vi "Car-Wash.vi"() -> ()   [LabVIEW 2017]
panel:
  out "Enum 2":enum16{"ECO", "DEL"}(ring)
  in  "Enum":enum16{"DEL", "ECO"}(ring)
  in  "MWP 2":bool
  in  "?":bool
  out "output cluster":cluster{bool, bool}
  in  "Economy Wash":bool
  in  "Deluxe Wash":bool
  in  "MWP":bool
  out "Vehicle Out of Position":bool=TRUE
  out "Air Dry":bool
  out "Clear Water Rinse":bool
  out "Main High Press. Wash":bool
  out "Soap Application":bool
  out "Under body Wash":bool
  in  "ADP":bool
  in  "UBW":bool
  # "AUTOMATED CAR WASH"
  # "Purchase Selection"
  # "Car Wash Indicators"
  # "Car Wash Simulation Switches"
  # "Underbody wash\nposition \nSwitch"
  # "Main Wash \nPosition \nSwitch"
  # "Air Dry\nPosition\nSwitch"
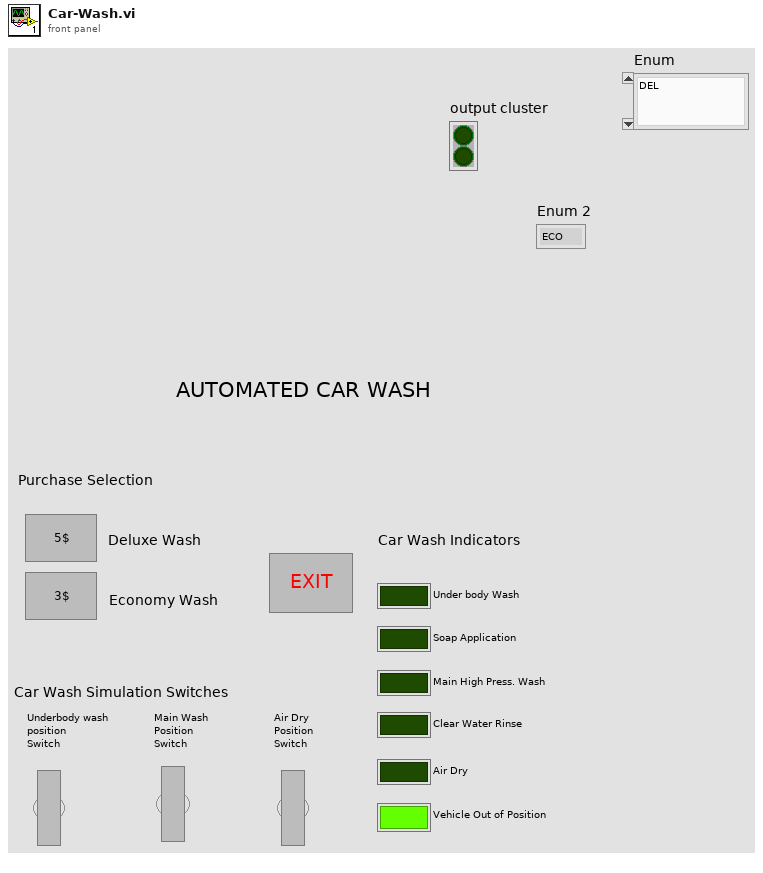
[diagram p1: front panel]
types:
  T1 = enum8{"Enabled", "Disabled", "Disabled and Grayed Out"}
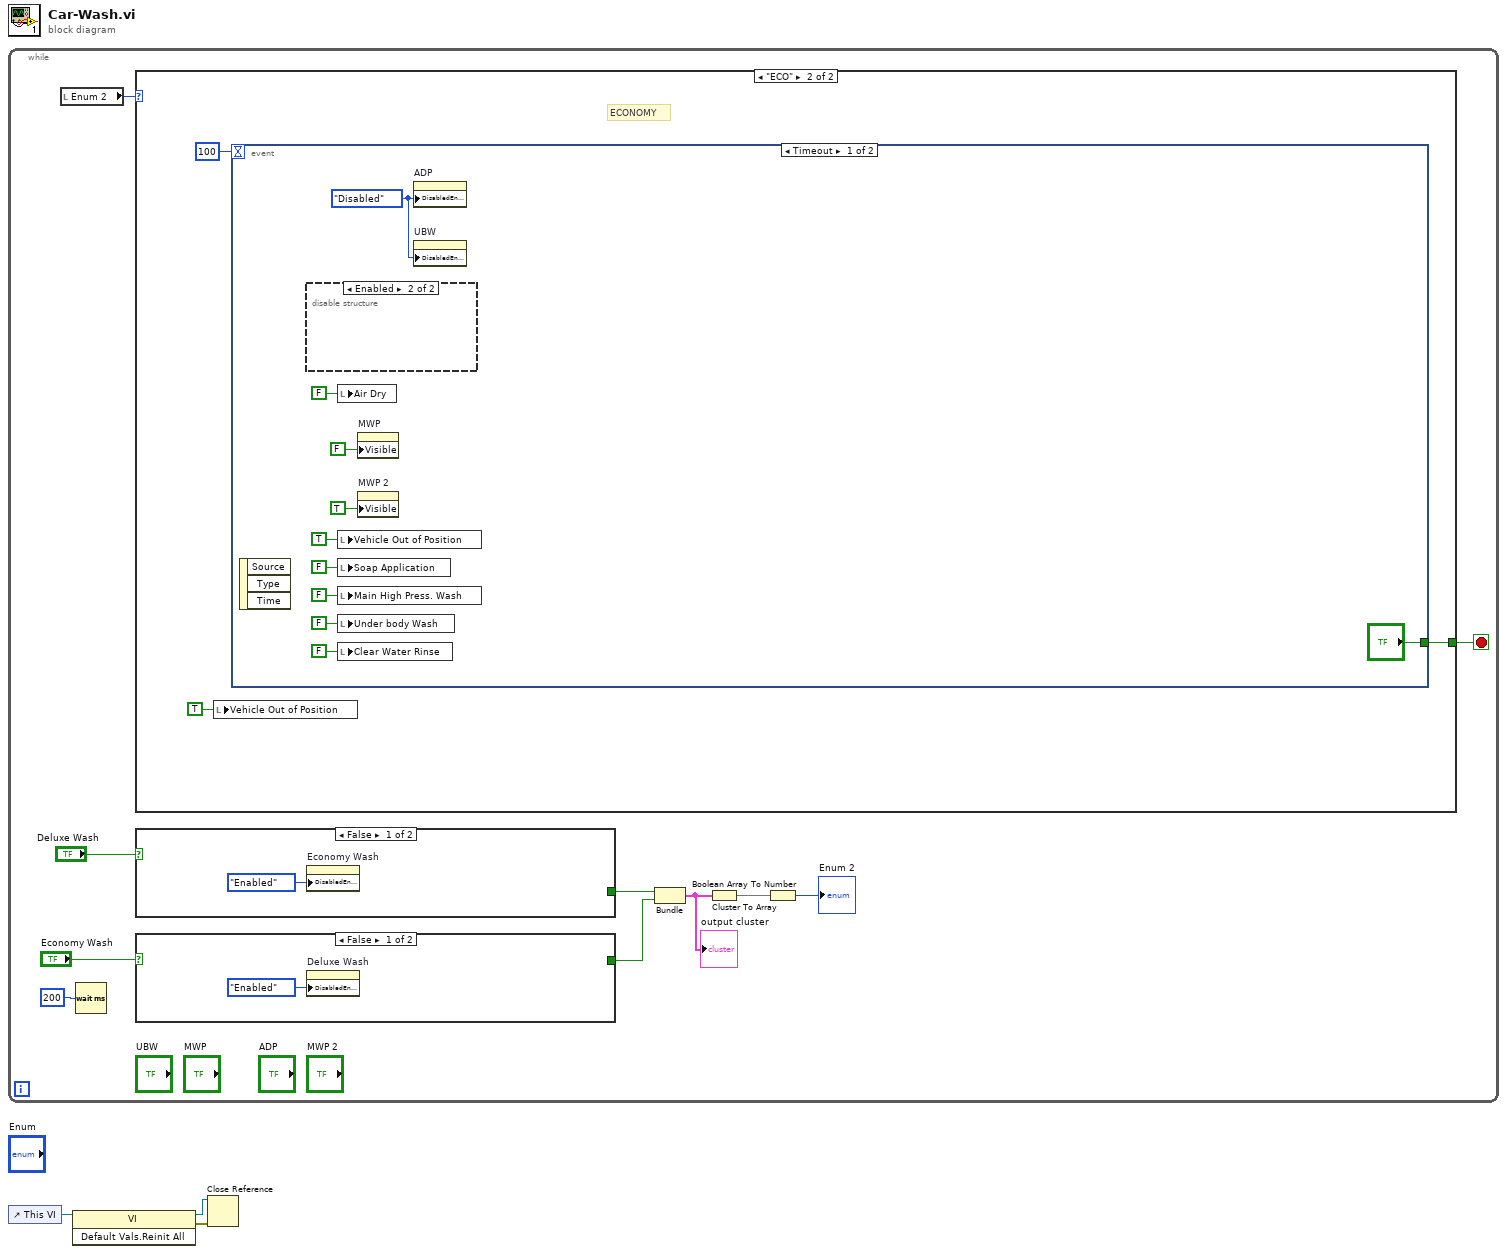
[diagram p0: block diagram]
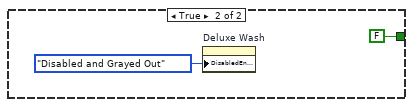
[diagram p2: hidden frame]
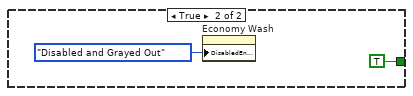
[diagram p3: hidden frame]
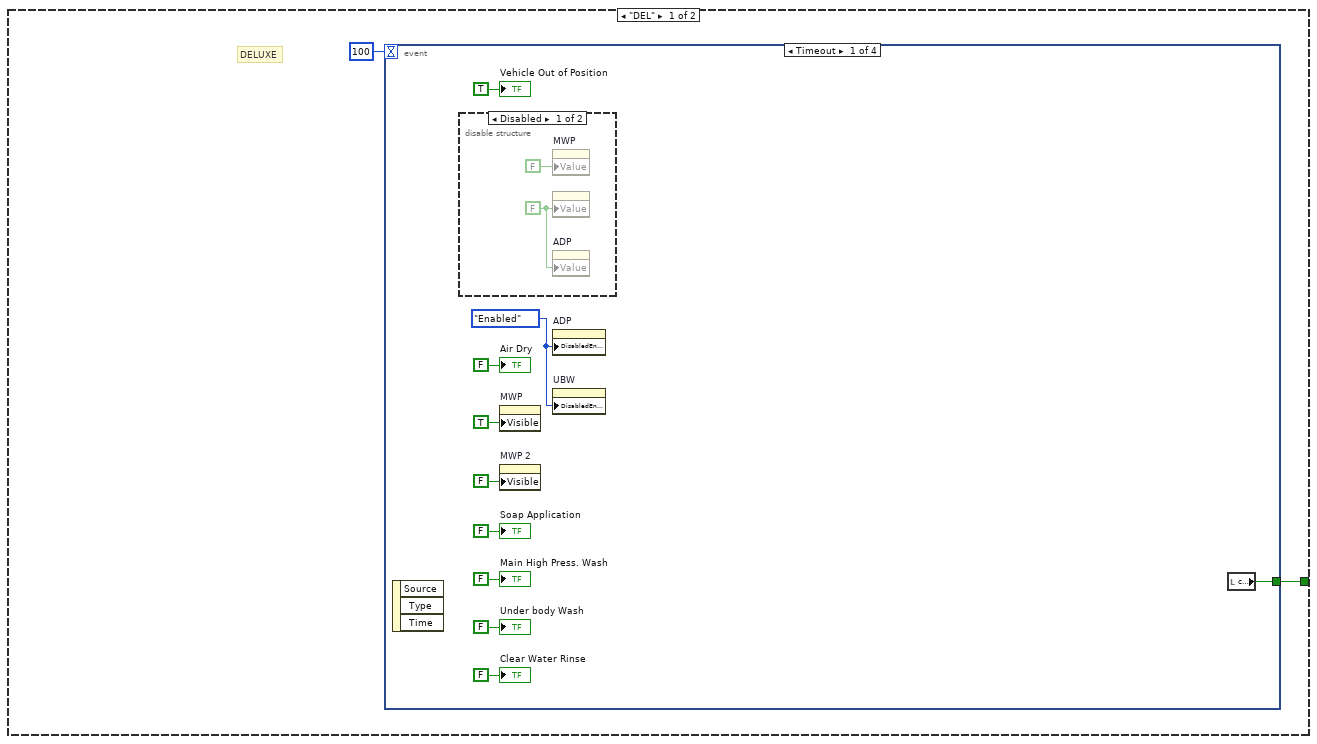
[diagram p4: hidden frame]
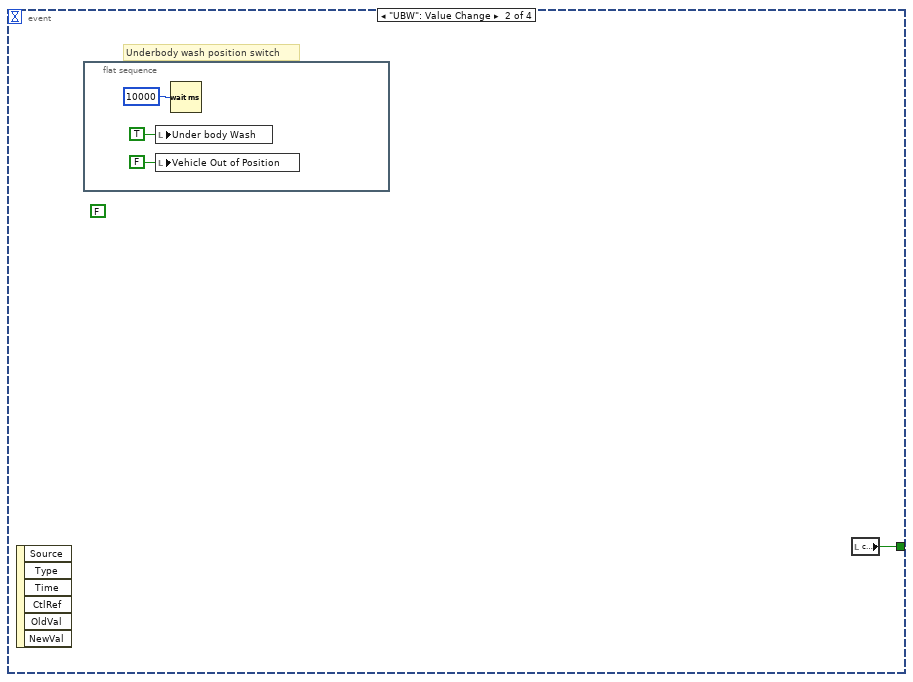
[diagram p6: hidden frame]
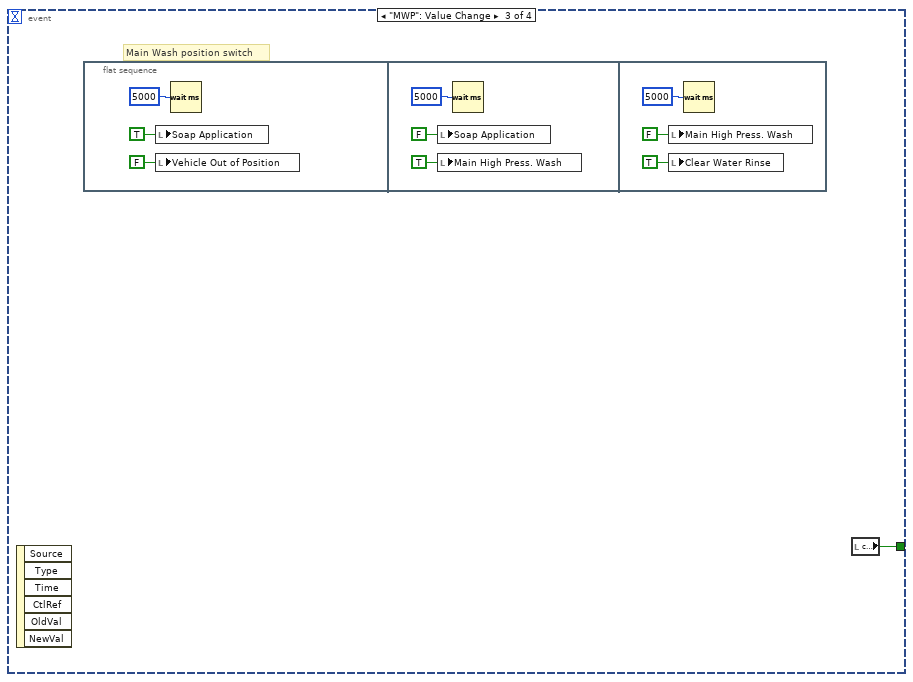
[diagram p7: hidden frame]
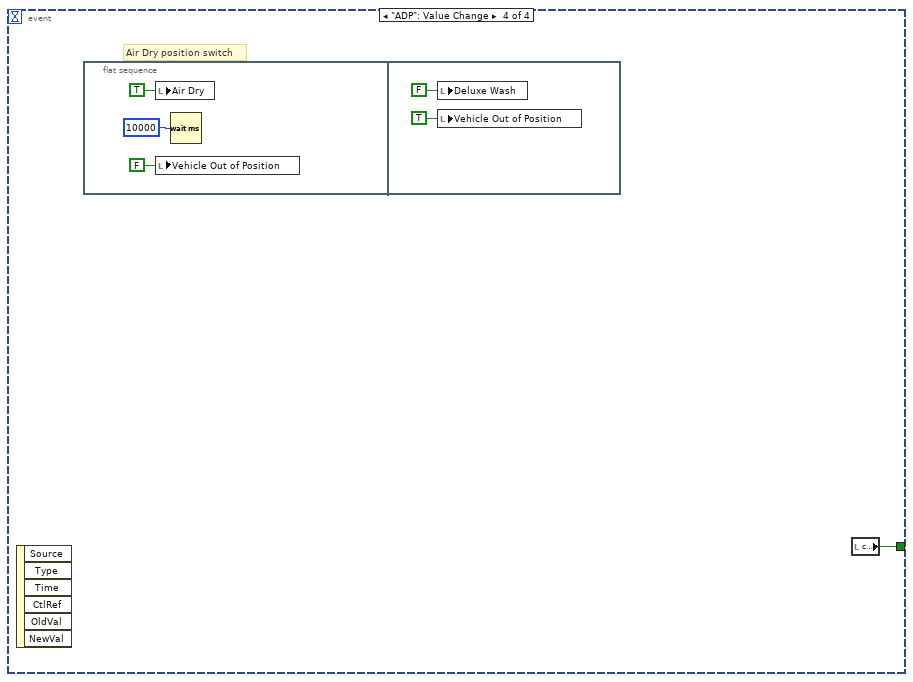
[diagram p8: hidden frame]
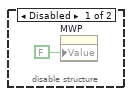
[diagram p9: hidden frame]
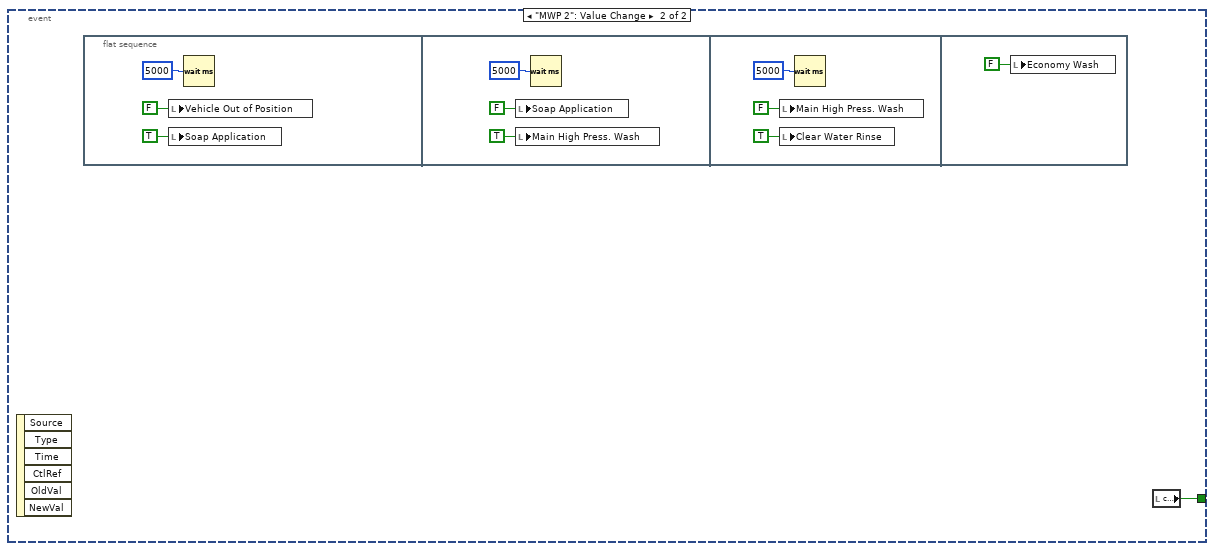
[diagram p10: hidden frame]
diagram:
  n1 = while {
    stop <- w12 stop-if-true
    n2 = local read "Enum 2"() -> (w4:enum16{"ECO", "DEL"})
    n3 = Wait (ms)(milliseconds to wait=u32 200) -> ()  [unwired: 1 out]
    n4 = case shown="\"ECO\"" w4 {
      tunnel: [w20 w54] -> w12
      frame "DEL" {
        # "DELUXE"
        n5 = event shown="[0] Timeout" {
          selector: _ -> [_ _ _ _]
          dyn-events: _ -> [_ _ _ _]
          timeout: 100 -> [_ _ _ _]
          tunnel: [w24 w34 w38 w48] -> w20
          event Timeout {
            w26 = T1."Enabled" ("Disabled")
            n6 = event-data() -> ()  [unwired: 1 in, 3 out]
            n7 = disable-structure shown="Disabled" {
              frame Disabled {
                w33 = FALSE
                n8 = property on="MWP" class="Bool"("Value"=FALSE) -> ()  [unwired: 2 in, 2 out]
                n9 = property on="UBW" class="Bool"("Value"=w33) -> ()  [unwired: 2 in, 2 out]
                n10 = property on="ADP" class="Bool"("Value"=w33) -> ()  [unwired: 2 in, 2 out]
              }
              frame Enabled {
              }
            }
            n11 = property on="MWP" class="Bool"("Visible"=TRUE) -> ()  [unwired: 2 in, 2 out]
            n12 = property on="MWP 2" class="Bool"("Visible"=FALSE) -> ()  [unwired: 2 in, 2 out]
            n13 = property on="ADP" class="Bool"("DisabledEnum"=w26) -> ()  [unwired: 2 in, 2 out]
            n14 = property on="UBW" class="Bool"("DisabledEnum"=w26) -> ()  [unwired: 2 in, 2 out]
            n15 = local read item#12() -> (w24:bool)
            "Air Dry" <- FALSE
            "Vehicle Out of Position" <- TRUE
            "Clear Water Rinse" <- FALSE
            "Under body Wash" <- FALSE
            "Main High Press. Wash" <- FALSE
            "Soap Application" <- FALSE
          }
          event "UBW": Value Change {
            (unwired) FALSE
            # "Underbody wash position switch"
            n16 = event-data() -> ()  [unwired: 1 in, 6 out]
            n17 = flat-sequence {
              frame #0 {
                n18 = local write "Under body Wash"(TRUE ("Under body Wash")) -> ()
                n19 = local write "Vehicle Out of Position"(FALSE ("Vehicle Out of Position")) -> ()
                n20 = Wait (ms)(milliseconds to wait=u32 10000) -> ()  [unwired: 1 out]
              }
            }
            n21 = local read item#12() -> (w34:bool)
          }
          event "MWP": Value Change {
            # "Main Wash position switch"
            n22 = event-data() -> ()  [unwired: 1 in, 6 out]
            n23 = flat-sequence {
              frame #0 {
                n24 = local write "Soap Application"(TRUE ("Air Dry")) -> ()
                n25 = local write "Vehicle Out of Position"(FALSE ("Vehicle Out of Position")) -> ()
                n26 = Wait (ms)(milliseconds to wait=u32 5000) -> ()  [unwired: 1 out]
              }
              frame #1 {
                n27 = local write "Soap Application"(FALSE ("Air Dry")) -> ()
                n28 = local write "Main High Press. Wash"(TRUE ("Vehicle Out of Position")) -> ()
                n29 = Wait (ms)(milliseconds to wait=u32 5000) -> ()  [unwired: 1 out]
              }
              frame #2 {
                n30 = local write "Main High Press. Wash"(FALSE ("Air Dry")) -> ()
                n31 = local write "Clear Water Rinse"(TRUE ("Vehicle Out of Position")) -> ()
                n32 = Wait (ms)(milliseconds to wait=u32 5000) -> ()  [unwired: 1 out]
              }
            }
            n33 = local read item#12() -> (w38:bool)
          }
          event "ADP": Value Change {
            # "Air Dry position switch"
            n34 = event-data() -> ()  [unwired: 1 in, 6 out]
            n35 = flat-sequence {
              frame #0 {
                n36 = local write "Air Dry"(TRUE ("Boolean 2")) -> ()
                n37 = local write "Vehicle Out of Position"(FALSE ("Vehicle Out of Position")) -> ()
                n38 = Wait (ms)(milliseconds to wait=u32 10000) -> ()  [unwired: 1 out]
              }
              frame #1 {
                n39 = local write "Deluxe Wash"(FALSE ("Deluxe Wash")) -> ()
                n40 = local write "Vehicle Out of Position"(TRUE ("Vehicle Out of Position")) -> ()
              }
            }
            n41 = local read item#12() -> (w48:bool)
          }
        }
      }
      frame "ECO" {
        # "ECONOMY"
        n42 = local write "Vehicle Out of Position"(TRUE ("Vehicle Out of Position")) -> ()
        n43 = event shown="[0] Timeout" {
          selector: _ -> [_ _]
          dyn-events: _ -> [_ _]
          timeout: 100 -> [_ _]
          tunnel: ["?" w68] -> w54
          event Timeout {
            w60 = T1."Disabled" ("Disabled")
            n44 = event-data() -> ()  [unwired: 1 in, 3 out]
            n45 = disable-structure shown="Enabled" {
              frame Disabled {
                n46 = property on="MWP" class="Bool"("Value"=FALSE ("MWP")) -> ()  [unwired: 2 in, 2 out]
              }
              frame Enabled {
              }
            }
            n47 = local write "Air Dry"(FALSE) -> ()
            n48 = local write "Vehicle Out of Position"(TRUE ("Vehicle Out of Position")) -> ()
            n49 = local write "Soap Application"(FALSE) -> ()
            n50 = local write "Main High Press. Wash"(FALSE) -> ()
            n51 = local write "Under body Wash"(FALSE) -> ()
            n52 = local write "Clear Water Rinse"(FALSE) -> ()
            n53 = property on="MWP" class="Bool"("Visible"=FALSE) -> ()  [unwired: 2 in, 2 out]
            n54 = property on="MWP 2" class="Bool"("Visible"=TRUE) -> ()  [unwired: 2 in, 2 out]
            n55 = property on="ADP" class="Bool"("DisabledEnum"=w60) -> ()  [unwired: 2 in, 2 out]
            n56 = property on="UBW" class="Bool"("DisabledEnum"=w60) -> ()  [unwired: 2 in, 2 out]
          }
          event "MWP 2": Value Change {
            n57 = event-data() -> ()  [unwired: 1 in, 6 out]
            n58 = flat-sequence {
              frame #0 {
                n59 = local write "Vehicle Out of Position"(FALSE ("Vehicle Out of Position")) -> ()
                n60 = local write "Soap Application"(TRUE ("Soap Application")) -> ()
                n61 = Wait (ms)(milliseconds to wait=u32 5000) -> ()  [unwired: 1 out]
              }
              frame #1 {
                n62 = local write "Soap Application"(FALSE ("Soap Application")) -> ()
                n63 = local write "Main High Press. Wash"(TRUE ("Main High Press. Wash")) -> ()
                n64 = Wait (ms)(milliseconds to wait=u32 5000) -> ()  [unwired: 1 out]
              }
              frame #2 {
                n65 = local write "Main High Press. Wash"(FALSE ("Main High Press. Wash")) -> ()
                n66 = local write "Clear Water Rinse"(TRUE ("Clear Water Rinse")) -> ()
                n67 = Wait (ms)(milliseconds to wait=u32 5000) -> ()  [unwired: 1 out]
              }
              frame #3 {
                n68 = local write "Economy Wash"(FALSE ("Economy Wash")) -> ()
              }
            }
            n69 = local read item#12() -> (w68:bool)
          }
        }
      }
    }
    n70 = case shown="False" "Deluxe Wash" {
      tunnel: [_ TRUE] -> w8
      frame False {
        n71 = property on="Economy Wash" class="Bool (strict)"("DisabledEnum"=T1."Enabled" ("Disabled")) -> ()  [unwired: 2 in, 2 out]
      }
      frame True {
        n72 = property on="Economy Wash" class="Bool (strict)"("DisabledEnum"=T1."Disabled and Grayed Out" ("Disabled")) -> ()  [unwired: 2 in, 2 out]
      }
    }
    n73 = case shown="False" "Economy Wash" {
      tunnel: [_ FALSE] -> w7
      frame False {
        n74 = property on="Deluxe Wash" class="Bool (strict)"("DisabledEnum"=T1."Enabled" ("Disabled")) -> ()  [unwired: 2 in, 2 out]
      }
      frame True {
        n75 = property on="Deluxe Wash" class="Bool (strict)"("DisabledEnum"=T1."Disabled and Grayed Out" ("Disabled")) -> ()  [unwired: 2 in, 2 out]
      }
    }
    n76 = Bundle(w8, w7) -> (w9:cluster{bool, bool})  [unwired: 1 in]
    "output cluster" <- w9
    n77 = Cluster To Array(cluster=w9) -> (array=w6:bool[])
    n78 = Boolean Array To Number(Boolean array=w6) -> (number=→"Enum 2":u16)
  }
  n79 = control-ref of="This VI"() -> (w3:refnum<vi>)
  n80 = invoke class="VI" method="Default Vals.Reinit All"(reference=w3) -> (reference out=w2:refnum<vi>, error out=w1:errorcluster)  [unwired: 2 in, 1 out]
  n81 = Close Reference(reference=w2, error in (no error)=w1) -> ()  [unwired: 1 out]
